vi "LED-ctrl ref scroll.vi"(9 "Single pass?":bool, 10 "LEDDisplay":refnum<vi>, 11 "String":string="The Software is the Instrument     ") -> ()   [LabVIEW 2011, in "LED Display.xctl"]
uses:
  LED Display.xctl
panel:
  # "This is the actual background task VI. It is reentrant and multiple clones of this VI may exist in memory, one for each of the LED XControls."
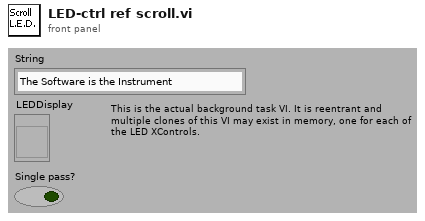
[diagram p1: front panel]
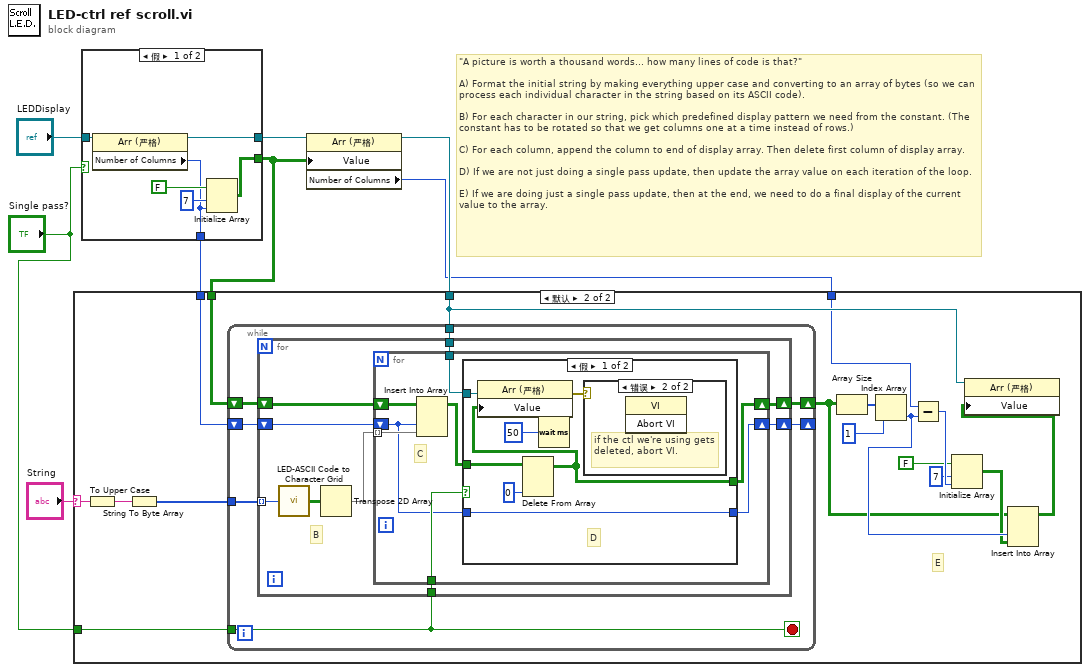
[diagram p0: block diagram]
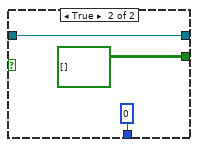
[diagram p2: hidden frame]
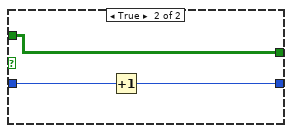
[diagram p5: hidden frame]
diagram:
  # "\"A picture is worth a thousand words... how many lines of code is that?\"\n\nA) Format the initial string by making everything upper case and converting to an array of bytes (so we can process each individual character in the string based on its ASCII code).\n\nB) For each character in our string, pick which predefined display pattern we need from the constant. (The constant has to be rotated so that we get columns one at a time instead of rows.)\n\nC) For each column, append the column to end of display array. Then delete first column of display array.\n\nD) If we are not just doing a single pass update, then update the array value on each iteration of the loop.\n\nE) If we are doing just a single pass update, then at the end, we need to do a final display of the current value to the array."
  n1 = case shown="假" "Single pass?" {
    tunnel: "LEDDisplay" -> [w14 w17]
    tunnel: [w13 w17] -> w6
    tunnel: [w12 bool[][] []] -> w5
    tunnel: [w9 u32 0 ("Number of Columns")] -> w2
    frame False {
      n2 = property class="Arr (严格)"(reference=w14) -> (reference out=w13:refnum<vi>, "Number of Columns"=w9:u32)  [unwired: 1 in, 1 out]
      n3 = Initialize Array(FALSE ("Boolean"), 7 ("dimension size"), w9) -> (w12:bool[][])
    }
    frame True {
    }
  }
  n4 = property class="Arr (严格)"(reference=w6, "Value"=w5) -> (reference out=w4:refnum<vi>, "Number of Columns"=w1:u32)  [unwired: 1 in, 1 out]
  n5 = case shown="默认" "String" {
    selector: "String" -> [_ w33]
    tunnel: w4 -> [_ w31]
    tunnel: w5 -> [_ w32]
    tunnel: "Single pass?" -> [_ w30]
    tunnel: w2 -> [_ w29]
    tunnel: w1 -> [_ w26]
    frame "" {
      # "do nothing for empty string."
    }
    frame Default {
      # "E"
      n6 = To Upper Case(1:w33) -> (0:w18:string)
      n7 = String To Byte Array(string=w18) -> (unsigned byte array=w34:u8[])
      n8 = while {
        tunnel: w34 -> [w41]
        shift-right: [w39] -> w20
        shift-left: w32 -> [w40]
        tunnel: w31 -> [w38]
        tunnel: w30 -> [w37]
        shift-right: [w35] -> _
        shift-left: w29 -> [w36]
        stop <- w37 stop-if-true
        n9 = for {
          shift-right: [w50] -> w39
          shift-left: w40 -> [w49]
          tunnel: w41 -> [w42] mode=indexing
          tunnel: w38 -> [w46]
          tunnel: w37 -> [w45]
          shift-right: [w43] -> w35
          shift-left: w36 -> [w44]
          # "B"
          n10 = call "LED-ASCII Code to Character Grid.vi"("ASCII Value"=w42) -> ("Character Grid"=w48:bool[][])
          n11 = Transpose 2D Array(2D array=w48) -> (transposed array=w47:bool[][])
          n12 = for {
            shift-right: [w53] -> w50
            shift-left: w49 -> [w56]
            tunnel: w47 -> [w55] mode=indexing
            tunnel: w46 -> [w58]
            tunnel: w45 -> [w57]
            shift-right: [w51] -> w43
            shift-left: w44 -> [w52]
            # "C"
            n13 = Insert Into Array(array=w56, index (col)=w52, new element=w55) -> (w54:bool[][])  [unwired: 1 in]
            n14 = case shown="假" w57 {
              tunnel: w58 -> [w64 _]
              tunnel: w54 -> [w61 w68]
              tunnel: [w60 w68] -> w53
              tunnel: w52 -> [w59 w67]
              tunnel: [w59 w66] -> w51
              frame False {
                # "D"
                n15 = Delete From Array(array=w61, index (col)=0 ("Disabled Index (col)")) -> (array with subset deleted=w60:bool[][])  [unwired: 2 in, 1 out]
                n16 = property class="Arr (严格)"(reference=w64, "Value"=w60) -> (error out=w63:errorcluster)  [unwired: 1 in, 1 out]
                n17 = Wait (ms)(milliseconds to wait=u32 50) -> ()  [unwired: 1 out]
                n18 = case shown="错误" w63 {
                  frame No Error {
                  }
                  frame Error {
                    # "if the ctl we're using gets deleted, abort VI."
                    n19 = invoke class="VI" method="Abort VI"() -> ()  [unwired: 3 in, 3 out]
                  }
                }
              }
              frame True {
                n20 = Increment(x=w67) -> (x+1=w66:u32)
              }
            }
          }
        }
      }
      n21 = Array Size(array=w20) -> (size(s)=w28:i32[])
      n22 = Index Array(array=w28, index=1) -> (element=w22:i32)
      n23 = Subtract(x=w26, y=w22) -> (x-y=w25:u32)
      n24 = Initialize Array(FALSE ("replace all? (F)"), 7 ("dimension size"), w25) -> (w21:bool[][])
      n25 = Insert Into Array(array=w20, index (col)=w22, new element=w21) -> (w19:bool[][])  [unwired: 1 in]
      n26 = property class="Arr (严格)"(reference=w31, "Value"=w19) -> ()  [unwired: 1 in, 2 out]
    }
  }
